vi "坐标计算.vi"(10 "网格大小":dbl, 11 "输入":cluster{"x":dbl, "y":dbl}) -> (3 "输出":cluster{"x":dbl, "y":dbl})   [LabVIEW 2012]
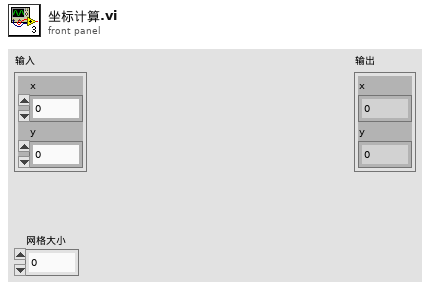
[diagram p1: front panel]
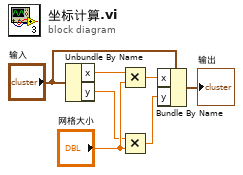
[diagram p0: block diagram]
diagram:
  n1 = Unbundle By Name("输入") -> ("x"=w5:dbl, "y"=w6:dbl)
  n2 = Multiply(x=w5, y="网格大小") -> (x*y=w4:dbl)
  n3 = Multiply(x=w6, y="网格大小") -> (x*y=w3:dbl)
  n4 = Bundle By Name(cluster="输入", "x"=w4, "y"=w3) -> (→"输出":cluster{"x":dbl, "y":dbl})
